vi "FGV Konfig Werte.vi"(0 "Auto Scale X":bool, 1 "Auto Scale Y":bool, 2 "X Anzeigedauer":T4 items=["5 min"=300, "10 min"=600, "15 min"=900, "20 min"=1200, "30 min"=1800, "45 min"=2700, "1 h"=3600], 3 "Y Anzeige MIN":T3 {"Y Anzeige MIN 6" format="%#_5g"; "Y Anzeige MIN 5" format="%#_5g"; "Y Anzeige MIN 4" format="%#_5g"; "Y Anzeige MIN 3" format="%#_5g"; "Y Anzeige MIN 2" format="%#_5g"; "Y Anzeige MIN 1" format="%#_5g"}, 4 "Y Anzeige MAX":T2 {"Y Anzeige MAX 6" format="%#_5g"; "Y Anzeige MAX 5" format="%#_5g"; "Y Anzeige MAX 4" format="%#_5g"; "Y Anzeige MAX 3" format="%#_5g"; "Y Anzeige MAX 2" format="%#_5g"; "Y Anzeige MAX 1" format="%#_5g"}, 5 "Werteanzeige":i32=2, 6 "Autoscale einzeln":bool[](array[boolean]), 7 "Mittelwertanzeige":bool, 8 "Referenzen":refnum<vi>[](array[refnum]), 9 "Aktionen":T5) -> (10 "Referenzen":refnum<vi>[](array[refnum]), 12 "Autoscale einzeln":bool[](array[boolean]), 13 "Mittelwertanzeige":bool, 14 "Auto Scale X":bool, 15 "Auto Scale Y":bool, 16 "X Anzeigedauer":T4 items=["5 min"=300, "10 min"=600, "15 min"=900, "20 min"=1200, "30 min"=1800, "45 min"=2700, "1 h"=3600], 17 "Y Anzeige MIN":T3 {"Y Anzeige MIN 6" format="%#_5g"; "Y Anzeige MIN 5" format="%#_5g"; "Y Anzeige MIN 4" format="%#_5g"; "Y Anzeige MIN 3" format="%#_5g"; "Y Anzeige MIN 2" format="%#_5g"; "Y Anzeige MIN 1" format="%#_5g"}, 18 "Y Anzeige MAX":T2 {"Y Anzeige MAX 6" format="%#_5g"; "Y Anzeige MAX 5" format="%#_5g"; "Y Anzeige MAX 4" format="%#_5g"; "Y Anzeige MAX 3" format="%#_5g"; "Y Anzeige MAX 2" format="%#_5g"; "Y Anzeige MAX 1" format="%#_5g"}, 19 "Werteanzeige":i32)   [LabVIEW 2020, in "Grafik.lvlib"]
uses:
  Grafik.lvlib
  Visualisierungs Elemente/Auswahlfeld.ctl
  Visualisierungs Elemente/Zahlen-Eingabefeld.ctl
  Aktionen Konfig Diagramme.ctl
  Messdaten/Aktionen FGV Messdaten.ctl
  Messdaten/Messdaten.lvlib
  Allgemein/allgemeine Sub-VIs.lvlib
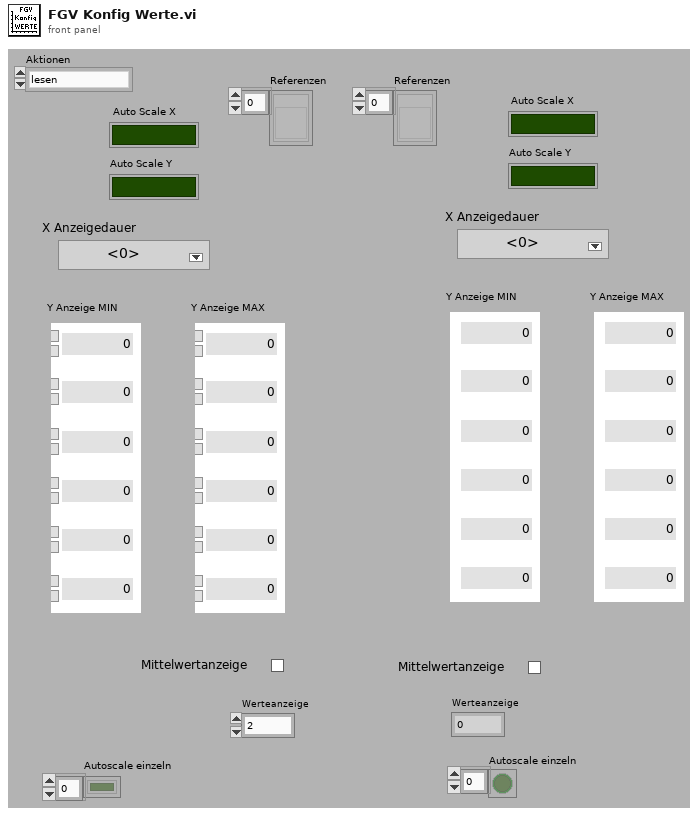
[diagram p1: front panel]
types:
  T1 = typedef "Zahlen-Eingabefeld.ctl" = sgl
  T2 = cluster{"Y Anzeige MAX 1":T1, "Y Anzeige MAX 2":T1, "Y Anzeige MAX 3":T1, "Y Anzeige MAX 4":T1, "Y Anzeige MAX 5":T1, "Y Anzeige MAX 6":T1}
  T3 = cluster{"Y Anzeige MIN 1":T1, "Y Anzeige MIN 2":T1, "Y Anzeige MIN 3":T1, "Y Anzeige MIN 4":T1, "Y Anzeige MIN 5":T1, "Y Anzeige MIN 6":T1}
  T4 = typedef "Auswahlfeld.ctl" = u16
  T5 = typedef "Grafik.lvlib/Aktionen Konfig Diagramme.ctl" = enum16{"lesen", "laden", "speichern", "X Auto Scale", "Y Auto Scale", "Anzeigedauer", "Y MIN", "Y MAX", "Referenzen", "Werteanzahl", "Autoscale einzeln"}
  T6 = typedef "Messdaten.lvlib/Aktionen FGV Messdaten.ctl" = enum16{"lesen", "schreiben", "löschen", "Mittelwerte", "Komponente"}
  T7 = cluster{"Auto Scale X":bool, "Auto Scale Y":bool, "X Anzeigedauer":T4, "Y Anzeige MIN":cluster{"Y Anzeige MIN 1":T1, "Y Anzeige MIN 2":T1, "Y Anzeige MIN 3":T1, "Y Anzeige MIN 4":T1, "Y Anzeige MIN 5":T1, "Y Anzeige MIN 6":T1}, "Y Anzeige MAX":cluster{"Y Anzeige MAX 1":T1, "Y Anzeige MAX 2":T1, "Y Anzeige MAX 3":T1, "Y Anzeige MAX 4":T1, "Y Anzeige MAX 5":T1, "Y Anzeige MAX 6":T1}, "Werteanzeige":i32, "Mittelwertanzeige":bool, "Autoscale einzeln":bool[]}
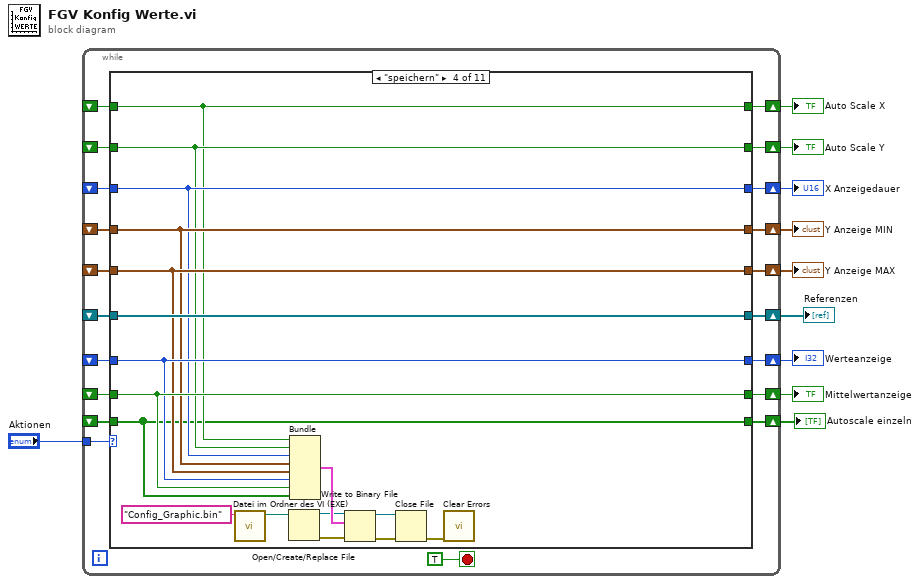
[diagram p0: block diagram]
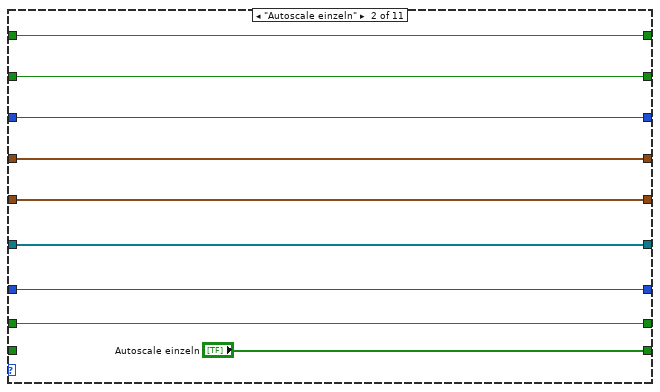
[diagram p3: hidden frame]
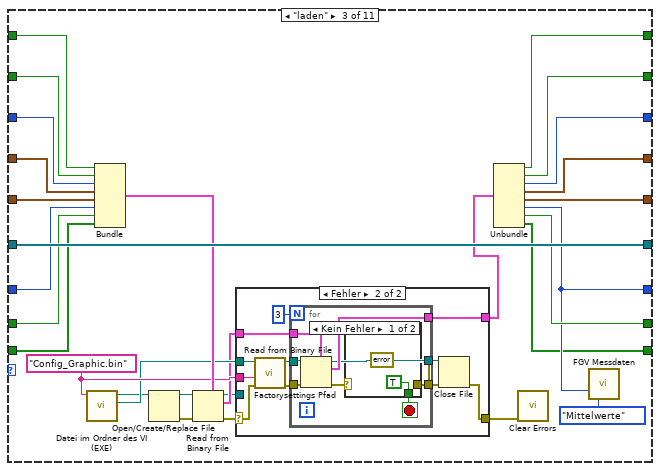
[diagram p4: hidden frame]
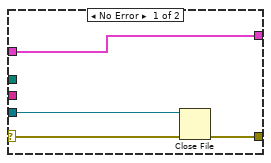
[diagram p5: hidden frame]
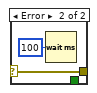
[diagram p6: hidden frame]
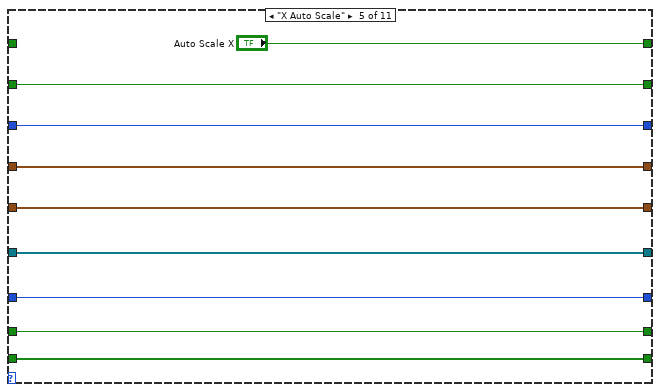
[diagram p7: hidden frame]
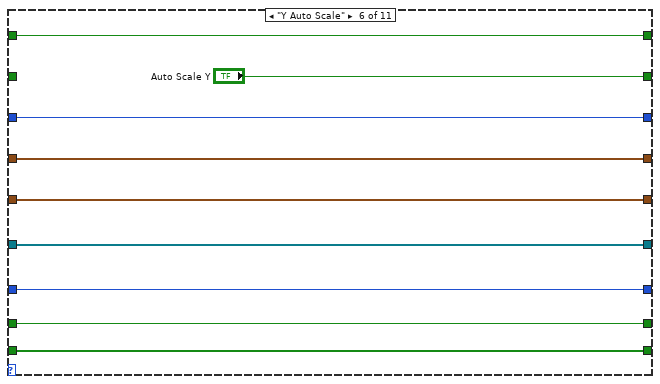
[diagram p8: hidden frame]
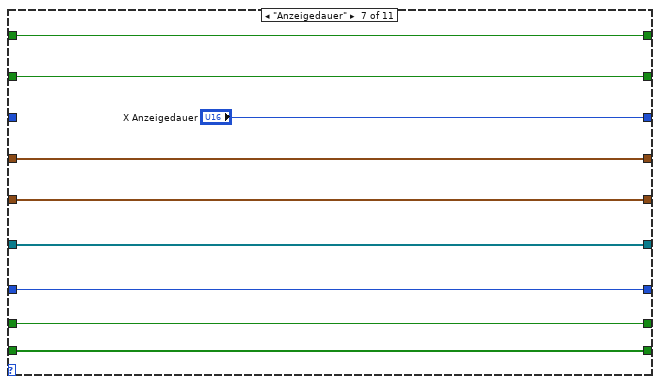
[diagram p9: hidden frame]
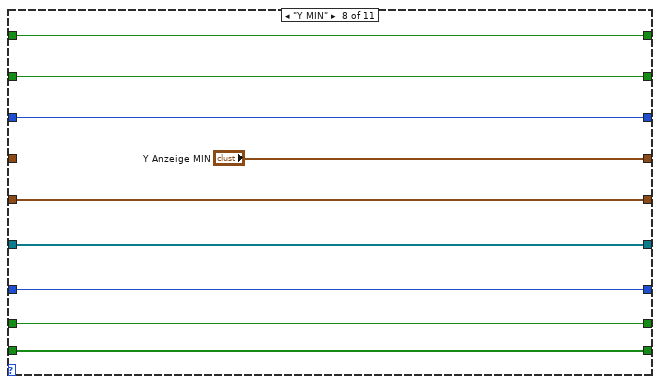
[diagram p10: hidden frame]
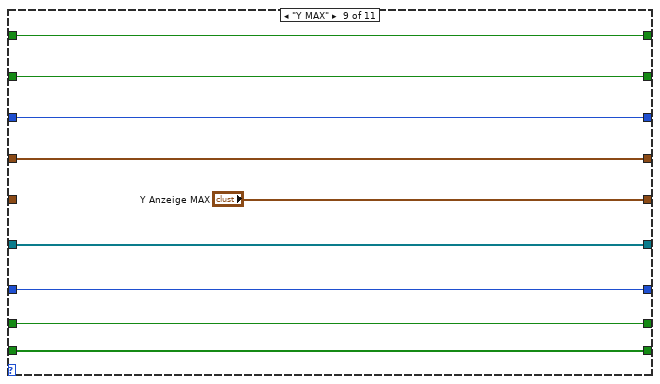
[diagram p11: hidden frame]
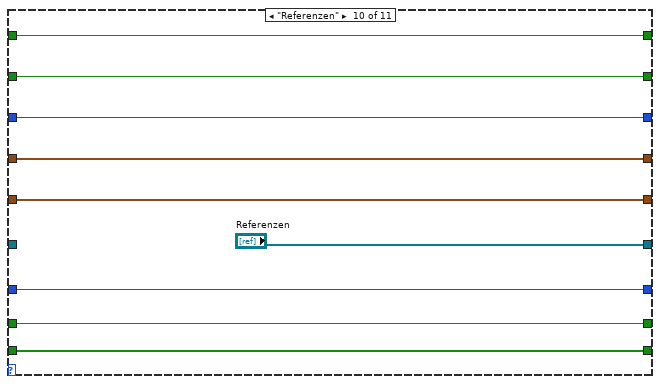
[diagram p12: hidden frame]
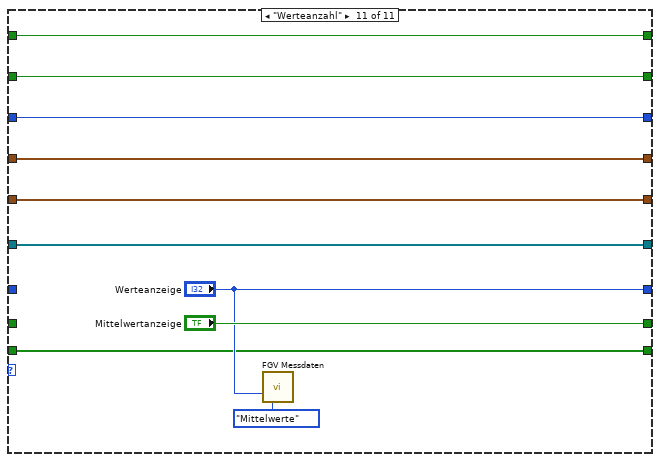
[diagram p13: hidden frame]
diagram:
  n1 = while {
    tunnel: "Aktionen" -> [w29]
    shift-right: [w19] -> w5
    shift-left: _ -> [w28]
    shift-right: [w20] -> w6
    shift-left: _ -> [w27]
    shift-right: [w21] -> w7
    shift-left: _ -> [w26]
    shift-right: [w22] -> w9
    shift-left: _ -> [w25]
    shift-right: [w23] -> w8
    shift-left: _ -> [w24]
    shift-right: [w18] -> w2
    shift-left: _ -> [w17]
    shift-right: [w16] -> w4
    shift-left: _ -> [w15]
    shift-right: [w14] -> w3
    shift-left: _ -> [w13]
    shift-right: [w12] -> w1
    shift-left: _ -> [w11]
    stop <- TRUE stop-if-true
    n2 = case shown="\"speichern\"" w29 {
      tunnel: w28 -> [w35 w44 w76 w114 _ w136 w145 w154 w163 w171 w185]
      tunnel: w27 -> [w36 w45 w75 w115 w127 _ w146 w155 w164 w172 w184]
      tunnel: w26 -> [w37 w46 w74 w116 w128 w137 _ w156 w165 w173 w183]
      tunnel: w25 -> [w38 w47 w73 w117 w129 w138 w147 _ w166 w174 w182]
      tunnel: w24 -> [w39 w48 w72 w118 w130 w139 w148 w157 _ w175 w181]
      tunnel: [w39 w48 w68 w118 w130 w139 w148 w157 "Y Anzeige MAX" w175 w181] -> w23
      tunnel: [w38 w47 w67 w117 w129 w138 w147 "Y Anzeige MIN" w166 w174 w182] -> w22
      tunnel: [w37 w46 w66 w116 w128 w137 "X Anzeigedauer" w156 w165 w173 w183] -> w21
      tunnel: [w36 w45 w65 w115 w127 "Auto Scale Y" w146 w155 w164 w172 w184] -> w20
      tunnel: [w35 w44 w64 w114 "Auto Scale X" w136 w145 w154 w163 w171 w185] -> w19
      tunnel: [w34 w43 w77 w121 w125 w134 w143 w152 w161 "Referenzen" w180] -> w18
      tunnel: w17 -> [w34 w43 w77 w121 w125 w134 w143 w152 w161 _ w180]
      tunnel: [w33 w42 w61 w119 w124 w133 w142 w151 w160 w170 "Werteanzeige"] -> w16
      tunnel: w15 -> [w33 w42 w71 w119 w124 w133 w142 w151 w160 w170 _]
      tunnel: [w32 w41 w63 w120 w123 w132 w141 w150 w159 w169 "Mittelwertanzeige"] -> w14
      tunnel: w13 -> [w32 w41 w70 w120 w123 w132 w141 w150 w159 w169 _]
      tunnel: [w31 "Autoscale einzeln" w59 w112 w122 w131 w140 w149 w158 w167 w176] -> w12
      tunnel: w11 -> [w31 _ w60 w112 w122 w131 w140 w149 w158 w167 w176]
      frame "lesen", Default {
      }
      frame "Autoscale einzeln" {
      }
      frame "laden" {
        w57 = "Config_Graphic.bin" ("Dateiname")
        n3 = call "Datei im Ordner des VI (EXE).vi"("Dateiname"=w57) -> ("Ordner des Haupt-VIs"=w56:path, "Dateipfad im Ordner des Haupt-VIs"=w51:path)  [unwired: 8 in, 1 out]
        n4 = Bundle("Auto Scale X"=w76, "Auto Scale Y"=w75, "X Anzeigedauer"=w74, "Y Anzeige MIN"=w73, "Y Anzeige MAX"=w72, "Werteanzeige"=w71, "Mittelwertanzeige"=w70, "Autoscale einzeln"=w60) -> (w69:T7)  [unwired: 1 in]
        n5 = Open/Create/Replace File(file path (use dialog)=w51) -> (refnum out=w50:refnum<file>, error out=w49:errorcluster)  [unwired: 5 in, 1 out]
        n6 = Read from Binary File(5:w69, 8:w49, 11:w50) -> (0:w58:errorcluster, 2:w55:T7, 3:w52:refnum<file>)  [unwired: 4 out]
        n7 = case shown="Fehler" w58 {
          selector: w58 -> [w80 w84]
          tunnel: w56 -> [_ w85]
          tunnel: w55 -> [w81 w83]
          tunnel: [w81 w91] -> w53
          tunnel: [w78 w89] -> w54
          tunnel: w52 -> [w79 _]
          tunnel: w57 -> [_ w82]
          frame No Error {
            n8 = Close File(refnum=w79, error in=w80) -> (error out=w78:errorcluster)  [unwired: 1 out]
          }
          frame Error {
            n9 = call "Factorysettings Pfad.vi"("error in (no error)"=w84, "Dateiname"=w82, "Ordner des Haupt-VIs"=w85) -> ("error out"=w86:errorcluster, "Pfad Factorysettings"=w87:path)  [unwired: 7 in]
            n10 = for {
              N: 3 -> [_]
              tunnel: w86 -> [w98]
              tunnel: w87 -> [w97]
              tunnel: [w96] -> w91
              tunnel: [w95] -> w90
              tunnel: [w94] -> w88
              tunnel: w83 -> [w93]
              stop <- w99 stop-if-true
              n11 = Read from Binary File(5:w93, 8:w98, 11:w97) -> (0:w100:errorcluster, 2:w96:T7, 3:w94:refnum<file>)  [unwired: 3 in, 1 out]
              n12 = case shown="Kein Fehler" w100 {
                selector: w100 -> [_ w103]
                tunnel: [TRUE _] -> w99
                tunnel: [errorcluster {"status"=FALSE, "code"=0, "source"=""} ("error IO") w103] -> w95
                frame No Error {
                }
                frame Error {
                  n13 = Wait (ms)(milliseconds to wait=u32 100 ("Zu wartende ms")) -> ()  [unwired: 1 out]
                }
              }
            }
            n14 = Close File(refnum=w88, error in=w90) -> (error out=w89:errorcluster)  [unwired: 1 out]
          }
        }
        n15 = Unbundle(w53) -> ("Auto Scale X"=w64:bool, "Auto Scale Y"=w65:bool, "X Anzeigedauer"=w66:T4, "Y Anzeige MIN"=w67:T3, "Y Anzeige MAX"=w68:T2, "Werteanzeige"=w61:i32, "Mittelwertanzeige"=w63:bool, "Autoscale einzeln"=w59:bool[])
        n16 = call <vilib>:"Clear Errors.vi"("error in (no error)"=w54) -> ()  [unwired: 5 in, 2 out]
        n17 = call "FGV Messdaten.vi"("Mittelwerte"=w61, "Aktionen"=Aktionen_FGV_Messdaten."Mittelwerte") -> ()  [unwired: 5 in, 9 out]
      }
      frame "speichern" {
        n18 = call "Datei im Ordner des VI (EXE).vi"("Dateiname"="Config_Graphic.bin") -> ("Dateipfad im Ordner des Haupt-VIs"=w110:path)  [unwired: 8 in, 2 out]
        n19 = Open/Create/Replace File(file path (use dialog)=w110) -> (refnum out=w108:refnum<file>, error out=w109:errorcluster)  [unwired: 5 in, 1 out]
        n20 = Bundle("Auto Scale X"=w114, "Auto Scale Y"=w115, "X Anzeigedauer"=w116, "Y Anzeige MIN"=w117, "Y Anzeige MAX"=w118, "Werteanzeige"=w119, "Mittelwertanzeige"=w120, "Autoscale einzeln"=w112) -> (w113:T7)  [unwired: 1 in]
        n21 = Write to Binary File(file (use dialog)=w108, data=w113, error in=w109) -> (refnum out=w106:refnum<file>, error out=w107:errorcluster)  [unwired: 4 out]
        n22 = Close File(refnum=w106, error in=w107) -> (error out=w105:errorcluster)  [unwired: 1 out]
        n23 = call <vilib>:"Clear Errors.vi"("error in (no error)"=w105) -> ()  [unwired: 5 in, 2 out]
      }
      frame "X Auto Scale" {
      }
      frame "Y Auto Scale" {
      }
      frame "Anzeigedauer" {
      }
      frame "Y MIN" {
      }
      frame "Y MAX" {
      }
      frame "Referenzen" {
      }
      frame "Werteanzahl" {
        n24 = call "FGV Messdaten.vi"("Mittelwerte"="Werteanzeige", "Aktionen"=Aktionen_FGV_Messdaten."Mittelwerte") -> ()  [unwired: 5 in, 9 out]
      }
    }
  }
  "Auto Scale Y" <- w6
  "Auto Scale X" <- w5
  "X Anzeigedauer" <- w7
  "Y Anzeige MAX" <- w8
  "Y Anzeige MIN" <- w9
  "Werteanzeige" <- w4
  "Mittelwertanzeige" <- w3
  "Referenzen" <- w2
  "Autoscale einzeln" <- w1
